vi "Calculate K and b.vi"(10 "X":dbl[](array[numeric]), 11 "Y":dbl[](array[numeric])) -> (2 "b":dbl, 3 "K":dbl)   [LabVIEW 2017, in "SQLite.lvclass"]
doc: "两点校准，计算K和b。\n2015-05-26 22:21:39\n蒋松\njiangsong@outlook.com"
uses:
  SQLite.lvclass
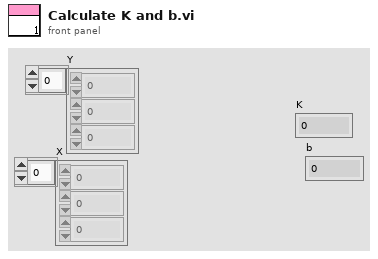
[diagram p1: front panel]
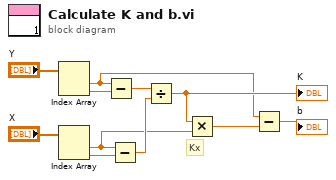
[diagram p0: block diagram]
diagram:
  # "Kx"
  n1 = Index Array(array="Y") -> (element #1=w3:dbl, element #2=w9:dbl)  [unwired: 2 in]
  n2 = Index Array(array="X") -> (element #1=w4:dbl, element #2=w8:dbl)  [unwired: 2 in]
  n3 = Subtract(x=w3, y=w9) -> (x-y=w7:dbl)
  n4 = Subtract(x=w4, y=w8) -> (x-y=w6:dbl)
  n5 = Divide(x=w7, y=w6) -> (x/y=w5:dbl)
  "K" <- w5
  n6 = Multiply(x=w5, y=w4) -> (x*y=w2:dbl)
  n7 = Subtract(x=w3, y=w2) -> (x-y=→"b":dbl)
